vi "Keithley 6514 Enable Status Registers.vi"(0 "Resource In":refnum<visa-resource-name>, 1 "Check For SCPI Errors? (T)":bool=TRUE, 5 "Register to Enable (Measurement)":u16(ring) items=["Measurement", "Operation", "Questionable"], 7 "Register Value":i32 min=0 max=65535 step=1 format="%016b", 11 "error in":T1) -> (4 "Resource Out":refnum<visa-resource-name>, 15 "error out":T1)   [LabVIEW 2014, in "KE6514Driver.lvlib"]
doc: "This VI is used to enable the various registers of the 6514.\n\nRegister to Set:\n0 = Measurement\n1 = Operation\n2 = Questionable\n\nRegister Value to Set:\n0 to 65535\nRefer to the Users Manual for complete description of the registers and associated bit values."
uses:
  KE6514Driver.lvlib
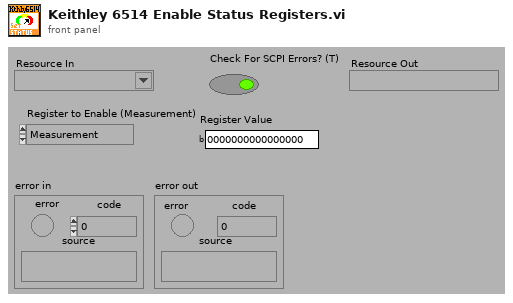
[diagram p1: front panel]
types:
  T1 = cluster{"error":bool, "code":i32, "source":string}
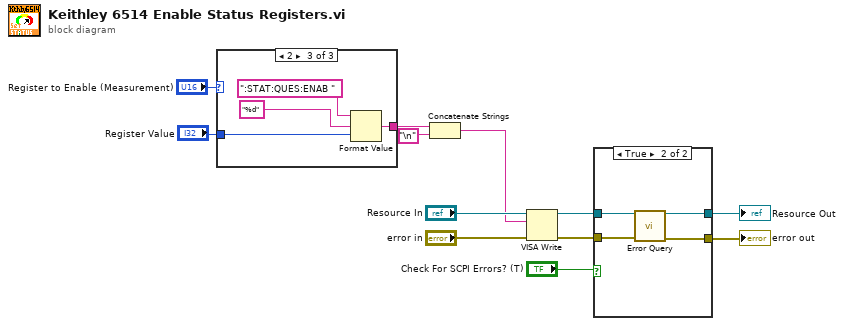
[diagram p0: block diagram]
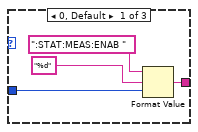
[diagram p3: hidden frame]
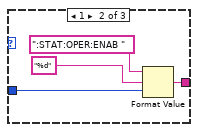
[diagram p4: hidden frame]
diagram:
  n1 = case shown="2" "Register to Enable (Measurement)" {
    tunnel: "Register Value" -> [w15 w19 w23]
    tunnel: [w13 w17 w21] -> w10
    frame 0, Default {
      n2 = Format Value(string ("")=":STAT:MEAS:ENAB ", format string="%d", value (0)=w15) -> (output string=w13:string)
    }
    frame 1 {
      n3 = Format Value(string ("")=":STAT:OPER:ENAB ", format string="%d", value (0)=w19) -> (output string=w17:string)
    }
    frame 2 {
      n4 = Format Value(string ("")=":STAT:QUES:ENAB ", format string="%d", value (0)=w23) -> (output string=w21:string)
    }
  }
  n5 = Concatenate Strings(w10, "\n") -> (w7:string)
  n6 = VISA Write(VISA resource name="Resource In", write buffer=w7, error in (no error)="error in") -> (VISA resource name out=w4:refnum<visa-resource-name>, error out=w3:errorcluster)  [unwired: 1 out]
  n7 = case shown="True" "Check For SCPI Errors? (T)" {
    tunnel: w4 -> [w26 w30]
    tunnel: w3 -> [w25 w29]
    tunnel: [w25 w28] -> w1
    tunnel: [w26 w27] -> w2
    frame False {
    }
    frame True {
      n8 = call "Error Query.vi"("VISA Resource In"=w30, "error in (no error)"=w29) -> ("VISA Resource Out (dupl)"=w27:refnum<visa-resource-name>, "error out"=w28:errorcluster)  [unwired: 10 in, 2 out]
    }
  }
  "error out" <- w1
  "Resource Out" <- w2
